vi "Reaffirm_ADAM_Outputs.vi"(3 "Channel Description":T1[](array[typedef]) {"Duty" format="%.0b"; "D" format="%#_5g"; "C" format="%#_5g"; "B" format="%#_5g"; "A" format="%#_5g"}, 4 "Active Ch Indicies":i32[](array[numeric]), 5 "Current Channel Values":dbl[](array[numeric]) format="%.2f") -> (1 "Scan Comments":string[](array[string]))   [LabVIEW 2012]
uses:
  ADAM Client/Sub VIs/ADAM Controls/Ch_description_ADAM.ctl
  ADAM Client/Sub VIs/ADAM Controls/Module_type_ADAM.ctl
  ADAM Client/Sub VIs/ADAM Controls/Function_ADAM.ctl
  ADAM Client/Sub VIs/ADAM Controls/Channel_State.ctl
  ADAM Client/Sub VIs/ADAM Controls/Calib_type_ADAM.ctl
  ADAM Client/Sub VIs/ADAM Controls/Address.ctl
  ADAM_Global.vi
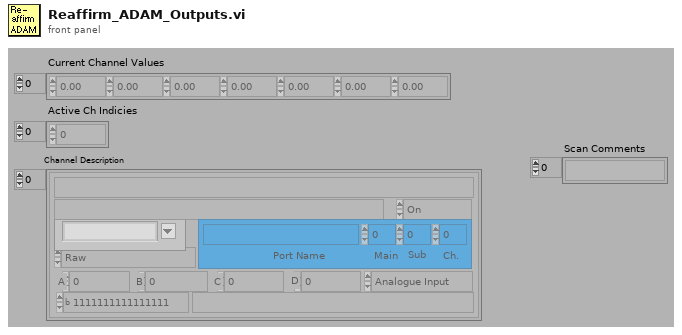
[diagram p1: front panel]
types:
  T1 = typedef "Ch_description_ADAM.ctl" = cluster{"Ch Name":string, "Type":T2, "Function":T3, "Ch State":T4, "Calibration type":T5, "A":dbl, "B":dbl, "C":dbl, "D":dbl, "Comments":string, "Address":T6, "String":string, "Duty":u16}
  T2 = typedef "Module_type_ADAM.ctl" = string
  T3 = typedef "Function_ADAM.ctl" = enum16{"Analogue Input", "Digital Input", "Event counter", "Event rate", "Analogue Output", "Digital Output", "Relay Output"}
  T4 = typedef "Channel_State.ctl" = enum16{"On", "Off", "Always On", "Always Off"}
  T5 = typedef "Calib_type_ADAM.ctl" = enum16{"Raw", "Bx + A", "Cx^2 + Bx + A", "Dx^3 + Cx^2 + Bx + A", "In Band", "Hi-Tec Q", "Hi-Tec M_dot", "Text"}
  T6 = typedef "Address.ctl" = cluster{"Main":i32, "Ch.":i32, "Sub":i32, "Port Name":string}
  T7 = typedef "Server_Control.ctl" = cluster{"Channel Name to control":string, "Channel sharing":enum16{"Channel Unshared", "Channel Shared by Rig", "Channel Shared by Group"}, "Default Value":dbl, "Client Array":string[], "Time Stamp":timestamp, "Do Not Reset":bool}
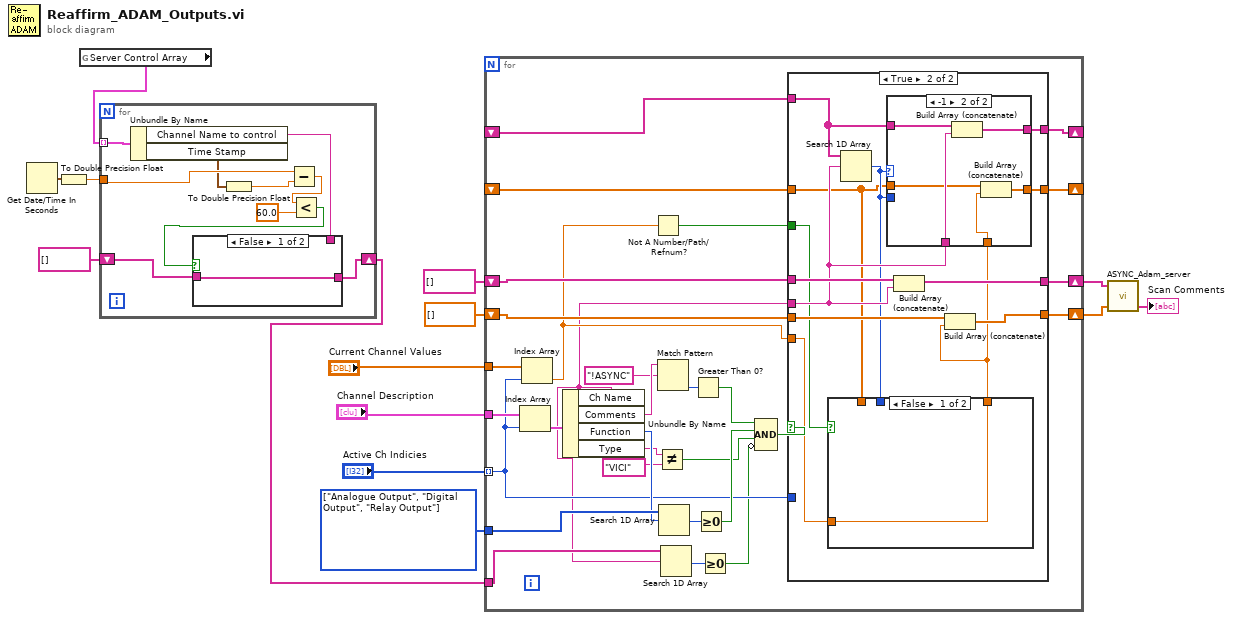
[diagram p0: block diagram]
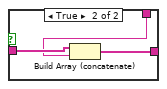
[diagram p2: hidden frame]
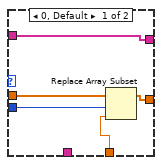
[diagram p4: hidden frame]
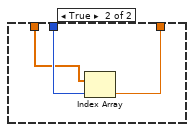
[diagram p5: hidden frame]
diagram:
  w12 = T3[] [enum."Analogue Output", enum."Digital Output", enum."Relay Output"] items=["Analogue Input", "Digital Input", "Event counter", "Event rate", "Analogue Output", "Digital Output", "Relay Output"]
  n1 = Get Date/Time In Seconds() -> (seconds since 1Jan1904=w4:timestamp)
  n2 = To Double Precision Float(number=w4) -> (double precision float=w3:dbl)
  n3 = global read "ADAM_Global.vi" "Server Control Array"() -> (w5:T7[])
  n4 = for {
    tunnel: w5 -> [w24] mode=indexing
    tunnel: w3 -> [w23]
    shift-right: [w16] -> w1
    shift-left: string[] [] -> [w17]
    n5 = Unbundle By Name(w24) -> ("Channel Name to control"=w15:string, "Time Stamp"=w22:timestamp)
    n6 = To Double Precision Float(number=w22) -> (double precision float=w21:dbl)
    n7 = Subtract(x=w23, y=w21) -> (x-y=w20:dbl)
    n8 = Less?(x=w20, y=60.0) -> (x < y?=w18:bool)
    n9 = case shown="False" w18 {
      tunnel: w17 -> [w25 w28]
      tunnel: [w25 w27] -> w16
      tunnel: w15 -> [_ w26]
      frame False {
      }
      frame True {
        n10 = Build Array (concatenate)(w28, w26) -> (w27:string[])
      }
    }
  }
  n11 = for {
    tunnel: "Channel Description" -> [w48]
    tunnel: "Active Ch Indicies" -> [w42] mode=indexing
    tunnel: w12 -> [w57]
    shift-right: [w46] -> w7
    shift-left: dbl[] [] -> [w47]
    shift-right: [w45] -> w8
    shift-left: string[] [] -> [w44]
    tunnel: "Current Channel Values" -> [w43]
    shift-right: [w37] -> _
    shift-left: _ -> [w38]
    shift-right: [w35] -> _
    shift-left: _ -> [w36]
    tunnel: w1 -> [w32]
    n12 = Index Array(array=w48, index=w42) -> (element=w58:T1)
    n13 = Index Array(array=w43, index=w42) -> (element=w34:dbl)
    n14 = Unbundle By Name(w58) -> ("Ch Name"=w31:string, "Comments"=w55:string, "Function"=w56:T3, "Type"=w41:T2)
    n15 = Not A Number/Path/Refnum?(number/path/refnum=w34) -> (NaN/Path/Refnum?=w33:bool)
    n16 = Not Equal?(x=w41, y=T2 "VICI" ("Type")) -> (x != y?=w39:bool)
    n17 = Match Pattern(string=w55, regular expression="!ASYNC") -> (offset past match=w53:i32)  [unwired: 4 out]
    n18 = Search 1D Array(1D array=w57, element=w56) -> (index of element=w52:i32)  [unwired: 1 out]
    n19 = Search 1D Array(1D array=w32, element=w31) -> (index of element=w30:i32)  [unwired: 1 out]
    n20 = Greater Than 0?(x=w53) -> (x > 0?=w50:bool)
    n21 = Greater Or Equal To 0?(x=w52) -> (x >= 0?=w51:bool)
    n22 = Greater Or Equal To 0?(x=w30) -> (x >= 0?=w29:bool)
    n23 = Compound Arithmetic op=AND(w50, w51, w39, invert w29) -> (w49:bool)
    n24 = case shown="True" w49 {
      tunnel: w42 -> [_ _]
      tunnel: w47 -> [w61 w75]
      tunnel: [w61 w74] -> w46
      tunnel: w31 -> [_ w70]
      tunnel: [w62 w73] -> w45
      tunnel: w44 -> [w62 w72]
      tunnel: w34 -> [_ w67]
      tunnel: w38 -> [w60 w71]
      tunnel: [w60 w69] -> w37
      tunnel: w36 -> [w59 w65]
      tunnel: [w59 w68] -> w35
      tunnel: w33 -> [_ w63]
      frame False {
      }
      frame True {
        n25 = Search 1D Array(1D array=w71, element=w70) -> (index of element=w66:i32)  [unwired: 1 out]
        n26 = case shown="False" w63 {
          tunnel: [w87 w88] -> w64
          tunnel: w67 -> [w87 _]
          tunnel: w66 -> [_ w90]
          tunnel: w65 -> [_ w89]
          frame False {
          }
          frame True {
            n27 = Index Array(array=w89, index=w90) -> (element=w88:dbl)
          }
        }
        n28 = case shown="-1" w66 {
          tunnel: w71 -> [w80 w86]
          tunnel: w70 -> [_ w85]
          tunnel: [w80 w84] -> w69
          tunnel: w66 -> [w79 _]
          tunnel: w65 -> [w78 w83]
          tunnel: [w77 w81] -> w68
          tunnel: w64 -> [w76 w82]
          frame 0, Default {
            n29 = Replace Array Subset(array=w78, new element=w76, index=w79) -> (w77:dbl[])
          }
          frame -1 {
            n30 = Build Array (concatenate)(w86, w85) -> (w84:string[])
            n31 = Build Array (concatenate)(w83, w82) -> (w81:dbl[])
          }
        }
        n32 = Build Array (concatenate)(w72, w70) -> (w73:string[])
        n33 = Build Array (concatenate)(w75, w64) -> (w74:dbl[])
      }
    }
  }
  n34 = call "ASYNC_Adam_server.vi"("Values"=w7, "Channel Names"=w8) -> ("Scan Comments"=→"Scan Comments":string[])  [unwired: 1 in, 2 out]
